vi "eyeballT2.vi"() -> ()   [LabVIEW 2018]
panel:
  in  "Numeric":i32
  out "error out":errorcluster
  in  "milliseconds to wait":u32
  out "Numeric 2":i32
  in  "stop":bool
  in  "error in (no error)":errorcluster
  in  "Python version":string="3.6"
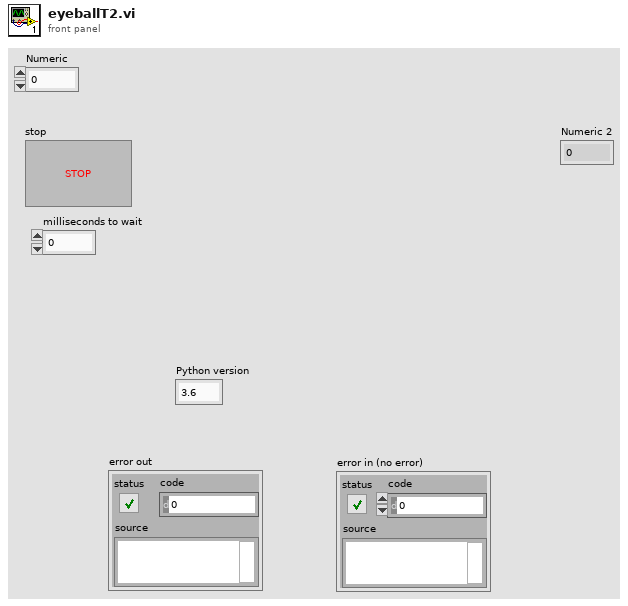
[diagram p1: front panel]
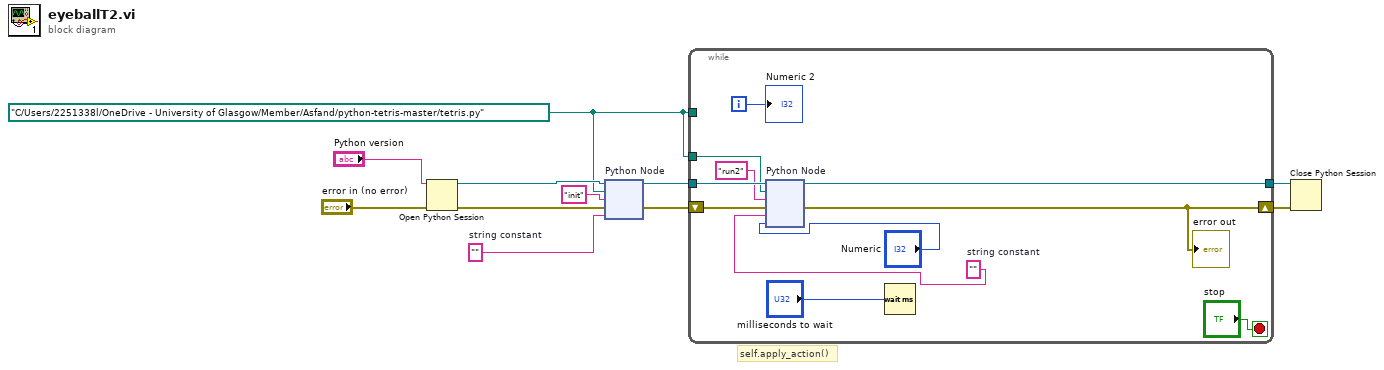
[diagram p0: block diagram]
diagram:
  w2 = path "C:/Users/2251338l/OneDrive - University of Glasgow/Member/Asfand/python-tetris-master/tetris.py" ("module path")
  w8 = ""  # string constant
  # "self.apply_action()"
  n1 = Open Python Session(python version="Python version", 3:"error in (no error)") -> (session out=w5:refnum<k35>, error out=w4:errorcluster)  [unwired: 1 in]
  n2 = node "Python Node"(w5, w2, "init" ("function name"), w4, w8) -> (w3:refnum<k35>, w1:errorcluster)  [unwired: 1 in, 2 out]
  n3 = while {
    shift-right: [w14] -> w6
    shift-left: w1 -> [w16]
    tunnel: w2 -> [_]
    tunnel: [w15] -> w7
    tunnel: w3 -> [w19]
    tunnel: w2 -> [w18]
    i -> [w21]
    stop <- "stop" stop-if-true
    w12 = ""  # string constant
    n4 = node "Python Node"(w19, w18, "run2" ("function name"), w16, w12, "Numeric") -> (w15:refnum<k35>, w14:errorcluster)  [unwired: 2 in, 2 out]
    "error out" <- w14
    n5 = Wait (ms)(milliseconds to wait="milliseconds to wait") -> ()  [unwired: 1 out]
    "Numeric 2" <- w21
  }
  n6 = Close Python Session(session in=w7, error in=w6) -> ()  [unwired: 1 out]
